vi "CreatMessageSection.vi"(0 "Port_No.":refnum<k21>, 2 "MessageFrame":refnum<k21>, 5 "错误输入（无错误）":errorcluster) -> (14 "session out":refnum<k21>, 15 "Sigs":refnum<k21>[](array[refnum]), 19 "error out":errorcluster)   [LabVIEW 2020]
uses:
  <vilib>/xnet/xnet.llb/XNET Create Session (Signal Output Single-point).vi
  <resource>/objmgr/xnet.rc
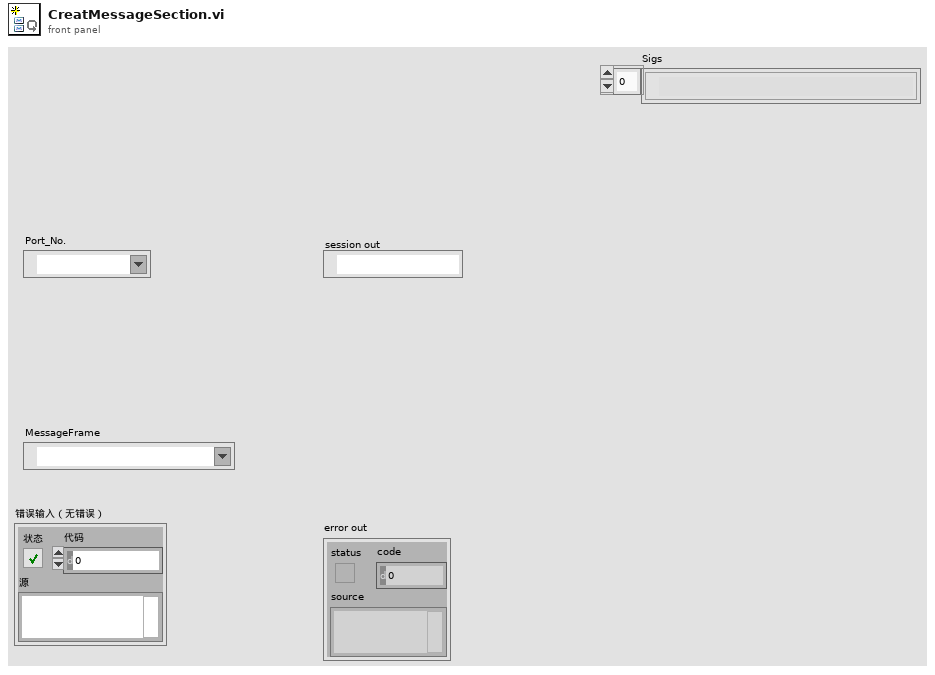
[diagram p1: front panel]
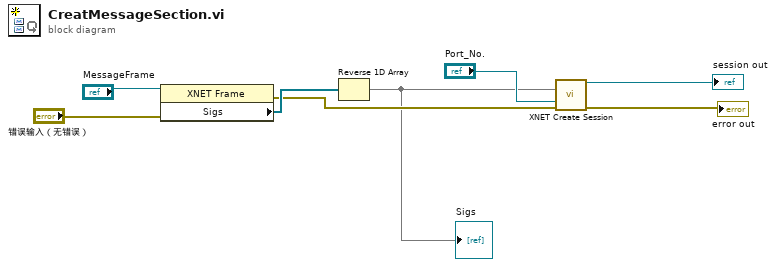
[diagram p0: block diagram]
diagram:
  n1 = property class="XNET Frame"(reference="MessageFrame", error in="错误输入（无错误）") -> (error out=w2:errorcluster, "Sigs"=w6:refnum<k21>[])  [unwired: 1 out]
  n2 = Reverse 1D Array(array=w6) -> (reversed array=w1:refnum<k21>[])
  "Sigs" <- w1
  n3 = call-poly <vilib>:"XNET Create Session.vi"("signal list"=w1, "interface"="Port_No.", "error in (no error)"=w2) -> ("session out"=→"session out":refnum<k21>, "error out"=→"error out":errorcluster)  [unwired: 11 out]
